vi "unflattenPressureFromXML_Array.vi"(8 "error in (no error)":errorcluster, 9 "pressureUnitInXML":T1, 10 "xmlString":string, 11 "pressureForType":dbl[unit][](array[numeric])=[26526.822968748813, 53053.645937497626, 79580.46890624643, 106107.29187499525]) -> (0 "error out":errorcluster, 3 "pressure":dbl[unit][](array[numeric]))   [LabVIEW 2012, in "UnitsAndXML.lvlib"]
uses:
  <userlib>/Common/UnitsAndXML/UnitsAndXML.lvlib
  <userlib>/Common/UnitsAndXML/FlattenItemWithUnitToXML/FlattenPressureToXML/PressureUnit.ctl
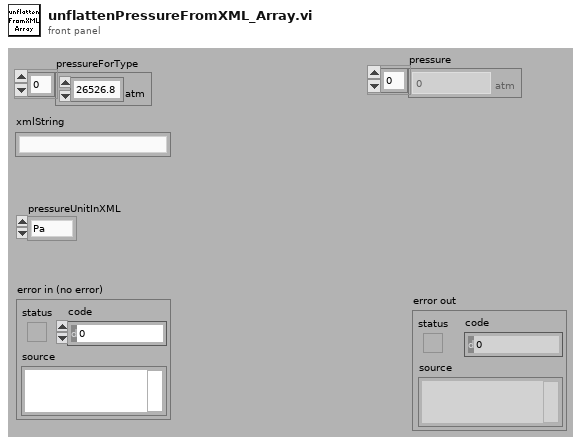
[diagram p1: front panel]
types:
  T1 = typedef "UnitsAndXML.lvlib/PressureUnit.ctl" = enum16{"Pa", "atm", "bar", "mbar", "m.Hg", "psi", "torr"}
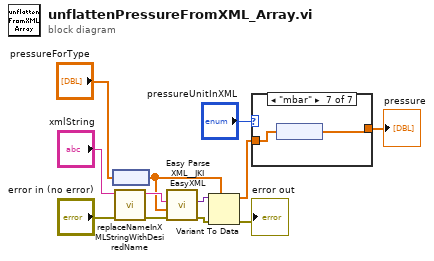
[diagram p0: block diagram]
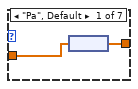
[diagram p2: hidden frame]
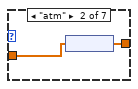
[diagram p3: hidden frame]
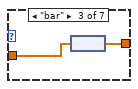
[diagram p4: hidden frame]
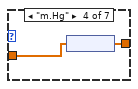
[diagram p5: hidden frame]
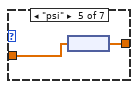
[diagram p6: hidden frame]
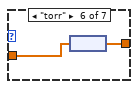
[diagram p7: hidden frame]
diagram:
  n1 = node("pressureForType") -> (w8:dbl[])
  n2 = call <userlib>:"replaceNameInXMLStringWithDesiredName.vi"("error in"="error in (no error)", "xmlString"="xmlString") -> ("error out"=w1:errorcluster, "revisedXMLString"=w9:string)  [unwired: 8 in]
  n3 = call <vilib>:"Easy Parse XML__JKI EasyXML.vi"("error in (no error)"=w1, "LabVIEW Data (Type)"=w8, "XML String"=w9) -> ("error out"=w4:errorcluster, "LabVIEW Data"=w11:variant)  [unwired: 7 in]
  n4 = Variant To Data(error in=w4, type=w8, Variant=w11) -> (data=w7:dbl[], error out=→"error out":errorcluster)
  n5 = case shown="\"mbar\"" "pressureUnitInXML" {
    tunnel: w7 -> [w13 w16 w18 w20 w22 w23 w26]
    tunnel: [w14 w15 w17 w19 w21 w24 w25] -> w6
    frame "Pa", Default {
      n6 = node(w13) -> (w14:dbl[unit][])
    }
    frame "atm" {
      n7 = node(w16) -> (w15:dbl[unit][])
    }
    frame "bar" {
      n8 = node(w18) -> (w17:dbl[unit][])
    }
    frame "m.Hg" {
      n9 = node(w20) -> (w19:dbl[unit][])
    }
    frame "psi" {
      n10 = node(w22) -> (w21:dbl[unit][])
    }
    frame "torr" {
      n11 = node(w23) -> (w24:dbl[unit][])
    }
    frame "mbar" {
      n12 = node(w26) -> (w25:dbl[unit][])
    }
  }
  "pressure" <- w6
